vi "Sel UnSel All.vi"(8 "error in (no error)":errorcluster, 10 "Check All? (T)":bool=TRUE, 11 "Methods ListCtrl":refnum<vi>) -> (0 "error out":errorcluster, 3 "Methods ListCtrl 2":refnum<vi>)   [LabVIEW 2020, in "WebServiceImporter.lvlib" / "Main Panel.lvlib" / "Select Methods.lvlib"]
uses:
  <vilib>/Platform/WebService/Main Panel/Pages/Select Methods/Select Methods.lvlib
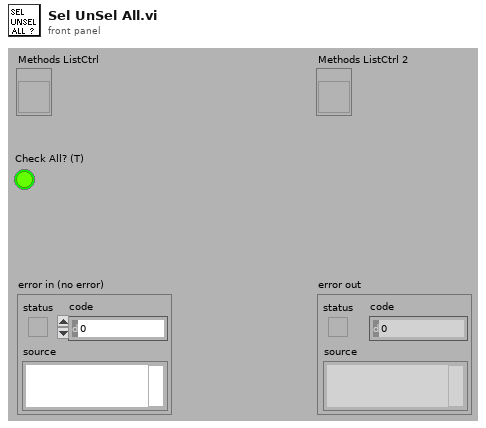
[diagram p1: front panel]
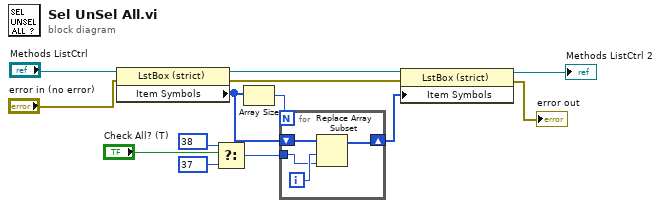
[diagram p0: block diagram]
diagram:
  n1 = property class="LstBox (strict)"(reference="Methods ListCtrl", error in="error in (no error)") -> (reference out=w9:refnum<vi>, error out=w7:errorcluster, "Item Symbols"=w4:i32[])
  n2 = Select(t=38, s="Check All? (T)", f=37) -> (s? t:f=w10:i32)
  n3 = Array Size(array=w4) -> (size(s)=w3:i32)
  n4 = for {
    N: w3 -> [_]
    tunnel: w10 -> [w15]
    shift-right: [w14] -> w8
    shift-left: w4 -> [w17]
    i -> [w16]
    n5 = Replace Array Subset(array=w17, new element=w15, index=w16) -> (w14:i32[])
  }
  n6 = property class="LstBox (strict)"(reference=w9, error in=w7, "Item Symbols"=w8) -> (reference out=→"Methods ListCtrl 2":refnum<vi>, error out=→"error out":errorcluster)
